vi "Read Aout Source.vi"(8 "error in (no error)":errorcluster, 11 "VISA resource name":refnum<visa-resource-name>) -> (0 "error out":errorcluster, 2 "aout source":cluster{"ASourceC":u16, "ASourceL":u16} {"ASourceL" items=["DEV", "BIAS", "GROUND"]; "ASourceC" items=["DEV", "BIAS", "GROUND"]}, 3 "VISA resource name out":refnum<visa-resource-name>)   [LabVIEW 2021, in "Andeen-Hagerling 2700A.lvlib"]
doc: "Each of the capacitance and loss analog outputs on the\nrear panel can be fed from any one of three internal sources;\nthe deviation subsystem, the bias voltage source, or the zero\nvoltage source. This VI returns which among these\nthree sources is connected to each of the rear panel analog\noutputs."
uses:
  Andeen-Hagerling 2700A.lvlib
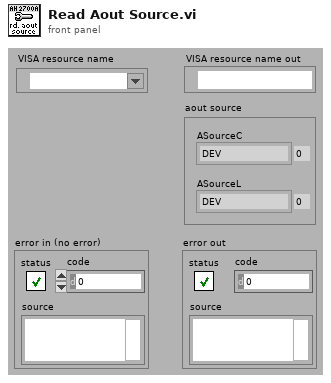
[diagram p1: front panel]
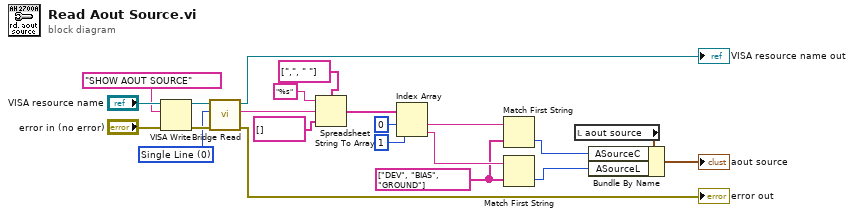
[diagram p0: block diagram]
diagram:
  w1 = u16 0 items=["Single Line", "Multi-Line"] ("Multiline")
  w5 = string[] ["DEV", "BIAS", "GROUND"]
  n1 = VISA Write(VISA resource name="VISA resource name", write buffer="SHOW AOUT SOURCE" ("command"), error in (no error)="error in (no error)") -> (VISA resource name out=w20:refnum<visa-resource-name>, error out=w19:errorcluster)  [unwired: 1 out]
  n2 = call "Bridge Read.vi"("error in (no error)"=w19, "multiline"=w1, "VISA resource name"=w20) -> ("error out"=→"error out":errorcluster, "read buffer"=w14:string, "VISA resource name out"=→"VISA resource name out":refnum<visa-resource-name>)  [unwired: 6 in]
  n3 = Spreadsheet String To Array(delimiter (Tab)=string[] [",", " "], format string="%s", spreadsheet string=w14, array type (2D Dbl)=string[] []) -> (array=w8:string[])
  n4 = Index Array(array=w8, index #1=0 ("index"), index #2=1 ("index")) -> (element #1=w7:string, element #2=w6:string)
  n5 = Match First String(2:w5, 3:w7) -> (0:w4:i32)  [unwired: 1 out]
  n6 = Match First String(2:w5, 3:w6) -> (0:w3:i32)  [unwired: 1 out]
  n7 = local read "aout source"() -> (w12:cluster{"ASourceC":u16, "ASourceL":u16})
  n8 = Bundle By Name(cluster=w12, "ASourceC"=w4, "ASourceL"=w3) -> (→"aout source":cluster{"ASourceC":u16, "ASourceL":u16})
